vi "Write Parameter File.vi"(8 "error in (no error)":errorcluster, 11 "CD Parameter Manager in":refnum<class "CD Parameter Manager.lvclass">) -> (0 "error out":errorcluster, 3 "CD Parameter Manager out":refnum<class "CD Parameter Manager.lvclass">)   [LabVIEW 2019, in "CD Parameter Manager API.lvlib" / "CD Parameter Manager.lvclass"]
uses:
  CD Parameter Manager.lvclass
  CD Parameter Manager.lvclass/CD Parameter Manager.ctl
  Parameter Generic File/Parameter Generic File.lvclass
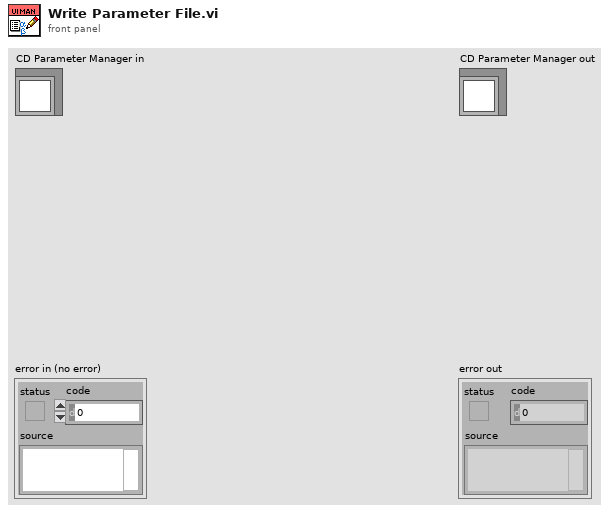
[diagram p1: front panel]
types:
  T1 = cluster{"Group name":string, "Controls":refnum<class "Parameter.lvclass">[]}[]
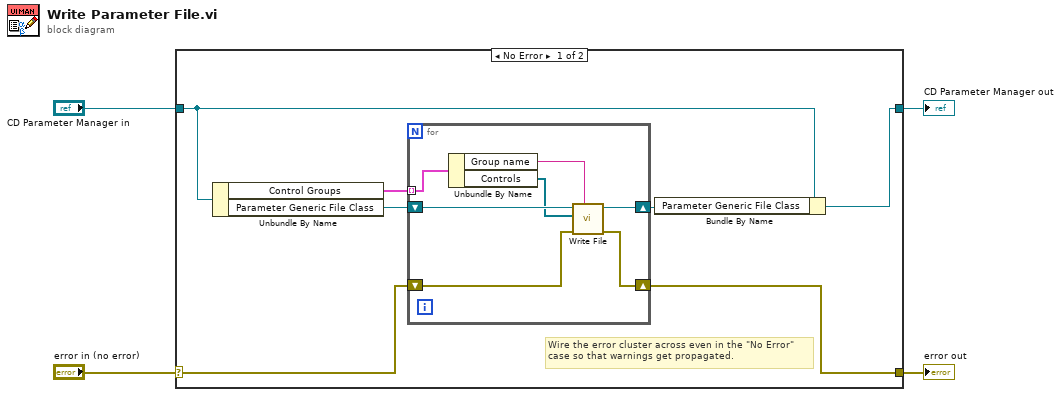
[diagram p0: block diagram]
diagram:
  n1 = case shown="No Error" "error in (no error)" {
    selector: "error in (no error)" -> [w11 w20]
    tunnel: [w10 w20] -> w3
    tunnel: [w6 w19] -> w1
    tunnel: "CD Parameter Manager in" -> [w7 w19]
    frame No Error {
      # "Wire the error cluster across even in the \"No Error\"\ncase so that warnings get propagated."
      n2 = Unbundle By Name(w7) -> ("Control Groups"=w5:T1, "Parameter Generic File Class"=w9:refnum<class "Parameter Generic File.lvclass">)
      n3 = for {
        shift-right: [w17] -> w10
        shift-left: w11 -> [w18]
        shift-right: [w15] -> w8
        shift-left: w9 -> [w16]
        tunnel: w5 -> [w14] mode=indexing
        n4 = Unbundle By Name(w14) -> ("Group name"=w12:string, "Controls"=w13:refnum<class "Parameter.lvclass">[])
        n5 = call-dynamic "Write File.vi"("Section"=w12, "error in (no error)"=w18, "Parameters"=w13, "Parameter Generic File in"=w16) -> ("error out"=w17:errorcluster, "Parameter Generic File out"=w15:refnum<class "Parameter Generic File.lvclass">)  [unwired: 6 in]
      }
      n6 = Bundle By Name(cluster=w7, "Parameter Generic File Class"=w8) -> (w6:refnum<class "CD Parameter Manager.lvclass">)
    }
    frame Error {
    }
  }
  "error out" <- w3
  "CD Parameter Manager out" <- w1
